vi "relativeListResultToAbsolute.vi"(11 "Dir-File Info Array":T1[](array[typedef])) -> (3 "Array":T1[](array[typedef]))   [LabVIEW 2017, in "_Try Beta Version of CSMF.lvlib"]
uses:
  _Try Beta Version of CSMF.lvlib
  FTP/controls/Dir-File Info.ctl
  FTP/controls/Dir-File Type.ctl
  FTP/FTP.lvclass
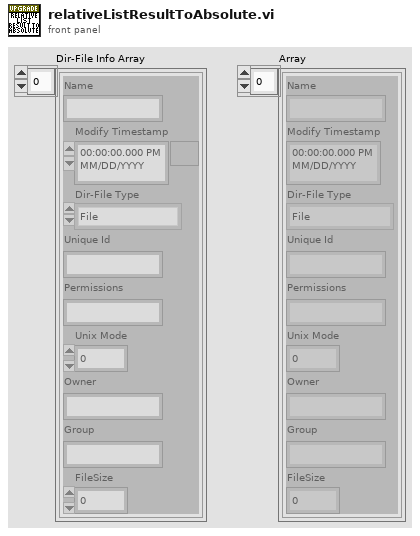
[diagram p1: front panel]
types:
  T1 = typedef "FTP_UpgradeCSMF.lvlib/FTP.lvclass/Dir-File Info.ctl" = cluster{"Name":string, "Modify Timestamp":timestamp, "Dir-File Type":T2, "Unique Id":string, "Permissions":string, "Unix Mode":u16, "Owner":string, "Group":string, "FileSize":i64}
  T2 = typedef "FTP_UpgradeCSMF.lvlib/FTP.lvclass/Dir-File Type.ctl" = enum16{"File", "Listed Directory", "Parent Directory", "Directory", "Unknown"}
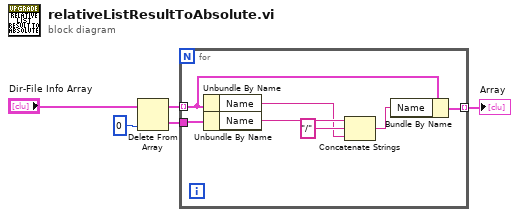
[diagram p0: block diagram]
diagram:
  n1 = Delete From Array(array="Dir-File Info Array", index=0) -> (deleted portion=w3:T1, array with subset deleted=w2:T1[])  [unwired: 1 in]
  n2 = for {
    tunnel: w2 -> [w8] mode=indexing
    tunnel: w3 -> [w12]
    tunnel: [w6] -> w5 mode=indexing
    n3 = Unbundle By Name(w8) -> ("Name"=w9:string)
    n4 = Unbundle By Name(w12) -> ("Name"=w11:string)
    n5 = Concatenate Strings(w11, "/" ("string"), w9) -> (w7:string)
    n6 = Bundle By Name(cluster=w8, "Name"=w7) -> (w6:T1)
  }
  "Array" <- w5
